vi "Interface Filter.vi"(8 "error in (no error)":errorcluster, 9 "Interface Filter":T5[](array[typedef]), 10 "fpga resources":T1[](array[typedef]) {"fpga cd" format="%.0x"}, 11 "Interface Names":string[](array[string])) -> (0 "error out":errorcluster, 3 "Compatible Interface Names":string[](array[string]))   [LabVIEW 2016, in "FPGA RM System Definition API.lvlib"]
uses:
  FPGA RM System Definition API.lvlib
  Shared/Requested Resource.ctl
  Types/Channel Type.ctl
  Types/resources.ctl
  <vilib>/NI Veristand/Custom Device API/Custom Device Item Ref.ctl
  Types/fpga resource.ctl
  Shared/FPGA RM Shared API.lvlib
  <vilib>/NI VeriStand/Custom Device API/Custom Device API.lvlib
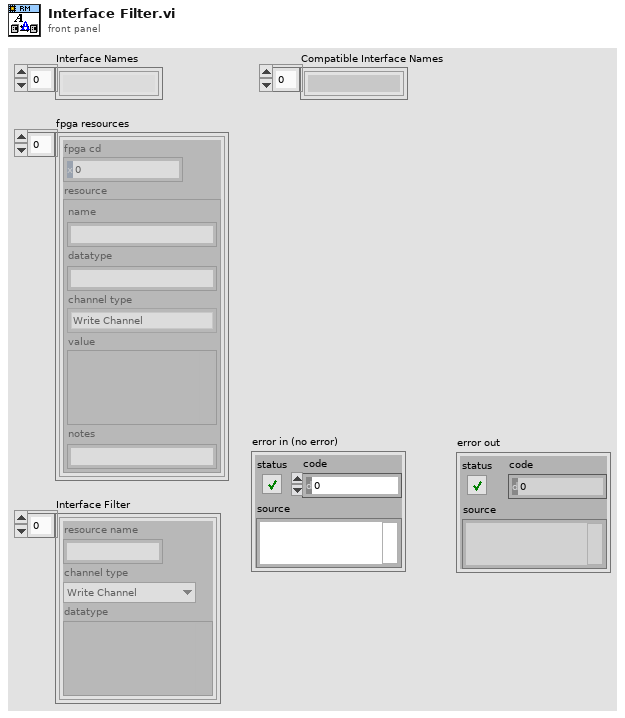
[diagram p1: front panel]
types:
  T1 = typedef "FPGA RM System Definition API.lvlib/resources.ctl" = cluster{"fpga cd":T2, "resource":T3}
  T2 = typedef "Custom Device API.lvlib/Custom Device Item Ref.ctl" = u64
  T3 = typedef "FPGA RM Shared API.lvlib/fpga resource.ctl" = cluster{"name":string, "datatype":string, "channel type":T4, "value":variant, "notes":string}
  T4 = typedef "FPGA RM Shared API.lvlib/Channel Type.ctl" = enum16{"Write Channel", "Read Channel", "Write Waveform", "Read Waveform"}
  T5 = typedef "FPGA RM Shared API.lvlib/Requested Resource.ctl" = cluster{"resource name":string, "channel type":T4, "datatype":variant}
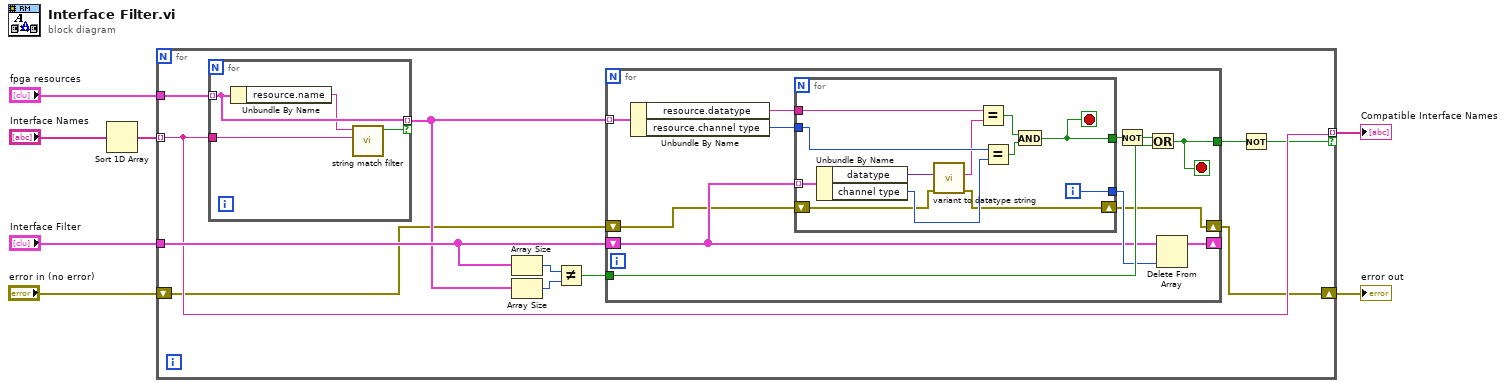
[diagram p0: block diagram]
diagram:
  n1 = Sort 1D Array(array="Interface Names") -> (sorted array=w5:string[])
  n2 = for {
    tunnel: "fpga resources" -> [w18]
    tunnel: w5 -> [w12] mode=indexing
    tunnel: "Interface Filter" -> [w17]
    tunnel: [w12] -> w7 mode=indexing if=w10
    shift-right: [w8] -> w1
    shift-left: "error in (no error)" -> [w9]
    n3 = for {
      tunnel: w18 -> [w45] mode=indexing
      tunnel: w12 -> [w46]
      tunnel: [w45] -> w16 mode=indexing if=w43
      n4 = Unbundle By Name(w45) -> ("resource.name"=w44:string)
      n5 = call "string match filter.vi"("string filter value"=w46, "string value"=w44) -> ("match?"=w43:bool)  [unwired: 9 in]
    }
    n6 = Array Size(array=w17) -> (size(s)=w14:i32)
    n7 = Array Size(array=w16) -> (size(s)=w15:i32)
    n8 = Not Equal?(x=w14, y=w15) -> (x != y?=w13:bool)
    n9 = for {
      tunnel: w16 -> [w30] mode=indexing
      tunnel: w13 -> [w25]
      tunnel: [w24] -> w11
      shift-right: [w21] -> _
      shift-left: w17 -> [w22]
      shift-right: [w19] -> w8
      shift-left: w9 -> [w20]
      stop <- w24 stop-if-true
      n10 = Unbundle By Name(w30) -> ("resource.datatype"=w29:string, "resource.channel type"=w28:T4)
      n11 = for {
        tunnel: w22 -> [w42] mode=indexing
        tunnel: w29 -> [w41]
        tunnel: w28 -> [w40]
        tunnel: [w36] -> w27
        tunnel: [w35] -> w23
        shift-right: [w31] -> w19
        shift-left: w20 -> [w32]
        i -> [w35]
        stop <- w36 stop-if-true
        n12 = Unbundle By Name(w42) -> ("datatype"=w34:variant, "channel type"=w39:T4)
        n13 = call "variant to datatype string.vi"("error in (no error)"=w32, "Variant"=w34) -> ("error out"=w31:errorcluster, "datatype string"=w33:string)  [unwired: 8 in]
        n14 = Equal?(x=w41, y=w33) -> (x = y?=w38:bool)
        n15 = Equal?(x=w40, y=w39) -> (x = y?=w37:bool)
        n16 = And(x=w38, y=w37) -> (x .and. y?=w36:bool)
      }
      n17 = Not(x=w27) -> (.not. x?=w26:bool)
      n18 = Or(x=w26, y=w25) -> (x .or. y?=w24:bool)
      n19 = Delete From Array(array=w22, index=w23) -> (array with subset deleted=w21:T5[])  [unwired: 1 in, 1 out]
    }
    n20 = Not(x=w11) -> (.not. x?=w10:bool)
  }
  "Compatible Interface Names" <- w7
  "error out" <- w1
